vi "test_csm_interface_descp.vi"() -> ()   [LabVIEW 2020]
uses:
  <userlib>/_NEVSTOP/Communicable State Machine(CSM)/_csmHelper/Typedef/Def-Argument Info.ctl
  4ae7eefc-6eeb-4361-9ef0-93d6dbb219bf.vi
  7e83fb4a-f3b1-4b26-86b0-b5537b9c493b.vi
  c018c89d-e81b-45ce-a165-17f998cd6f52.vi
  0c561034-f44a-4e92-a6ab-5fccff993fa6.vi
  <userlib>/_NEVSTOP/Communicable State Machine(CSM)/_Support/Common/Format Timestamp.vi
  <userlib>/_NEVSTOP/Communicable State Machine(CSM)/AdvanceAPI/CSM - Break Down Multiple States String.vi
  <userlib>/_NEVSTOP/Communicable State Machine(CSM)/AdvanceAPI/CSM - Compact Multiple States.vi
  <userlib>/_NEVSTOP/Communicable State Machine(CSM)/AdvanceAPI/CSM - Keywords.vi
  <userlib>/_NEVSTOP/Communicable State Machine(CSM)/addons/MassData-Parameter/_support/FGV-MassData(lvlibp).vi
  <userlib>/_NEVSTOP/Communicable State Machine(CSM)/addons/API-String-Arugments-Support/_Support/Convert API String Arguments to Data(variant).vi
  <userlib>/_NEVSTOP/Communicable State Machine(CSM)/_Shared/Trim Single-line Text.vi
  <userlib>/_NEVSTOP/Communicable State Machine(CSM)/_csmHelper/API/Create From VI Reference.vi
  <userlib>/_NEVSTOP/Communicable State Machine(CSM)/_csmHelper/API/Get All API Interface Info.vi
  <userlib>/_NEVSTOP/Communicable State Machine(CSM)/_csmHelper/API/Get All Status Interface Info.vi
  <userlib>/_NEVSTOP/Communicable State Machine(CSM)/_csmHelper/API/Destroy.vi
  <userlib>/_NEVSTOP/Communicable State Machine(CSM)/_csmHelper/CSM-Helper.lvclass
  <userlib>/_NEVSTOP/Communicable State Machine(CSM)/Communicable State Machine.lvlib
  _support/CSM Mermaid Support.lvlib
panel:
  out "ms":u32
  out "Array 4":cluster{string, "Argument":T1}[](array[cluster])
  out "Array":string[](array[string])
  out "resulting string":string
  out "State History":string
  out "Array 3":cluster{string, "Array":T1[], "Response":T1[]}[](array[cluster])
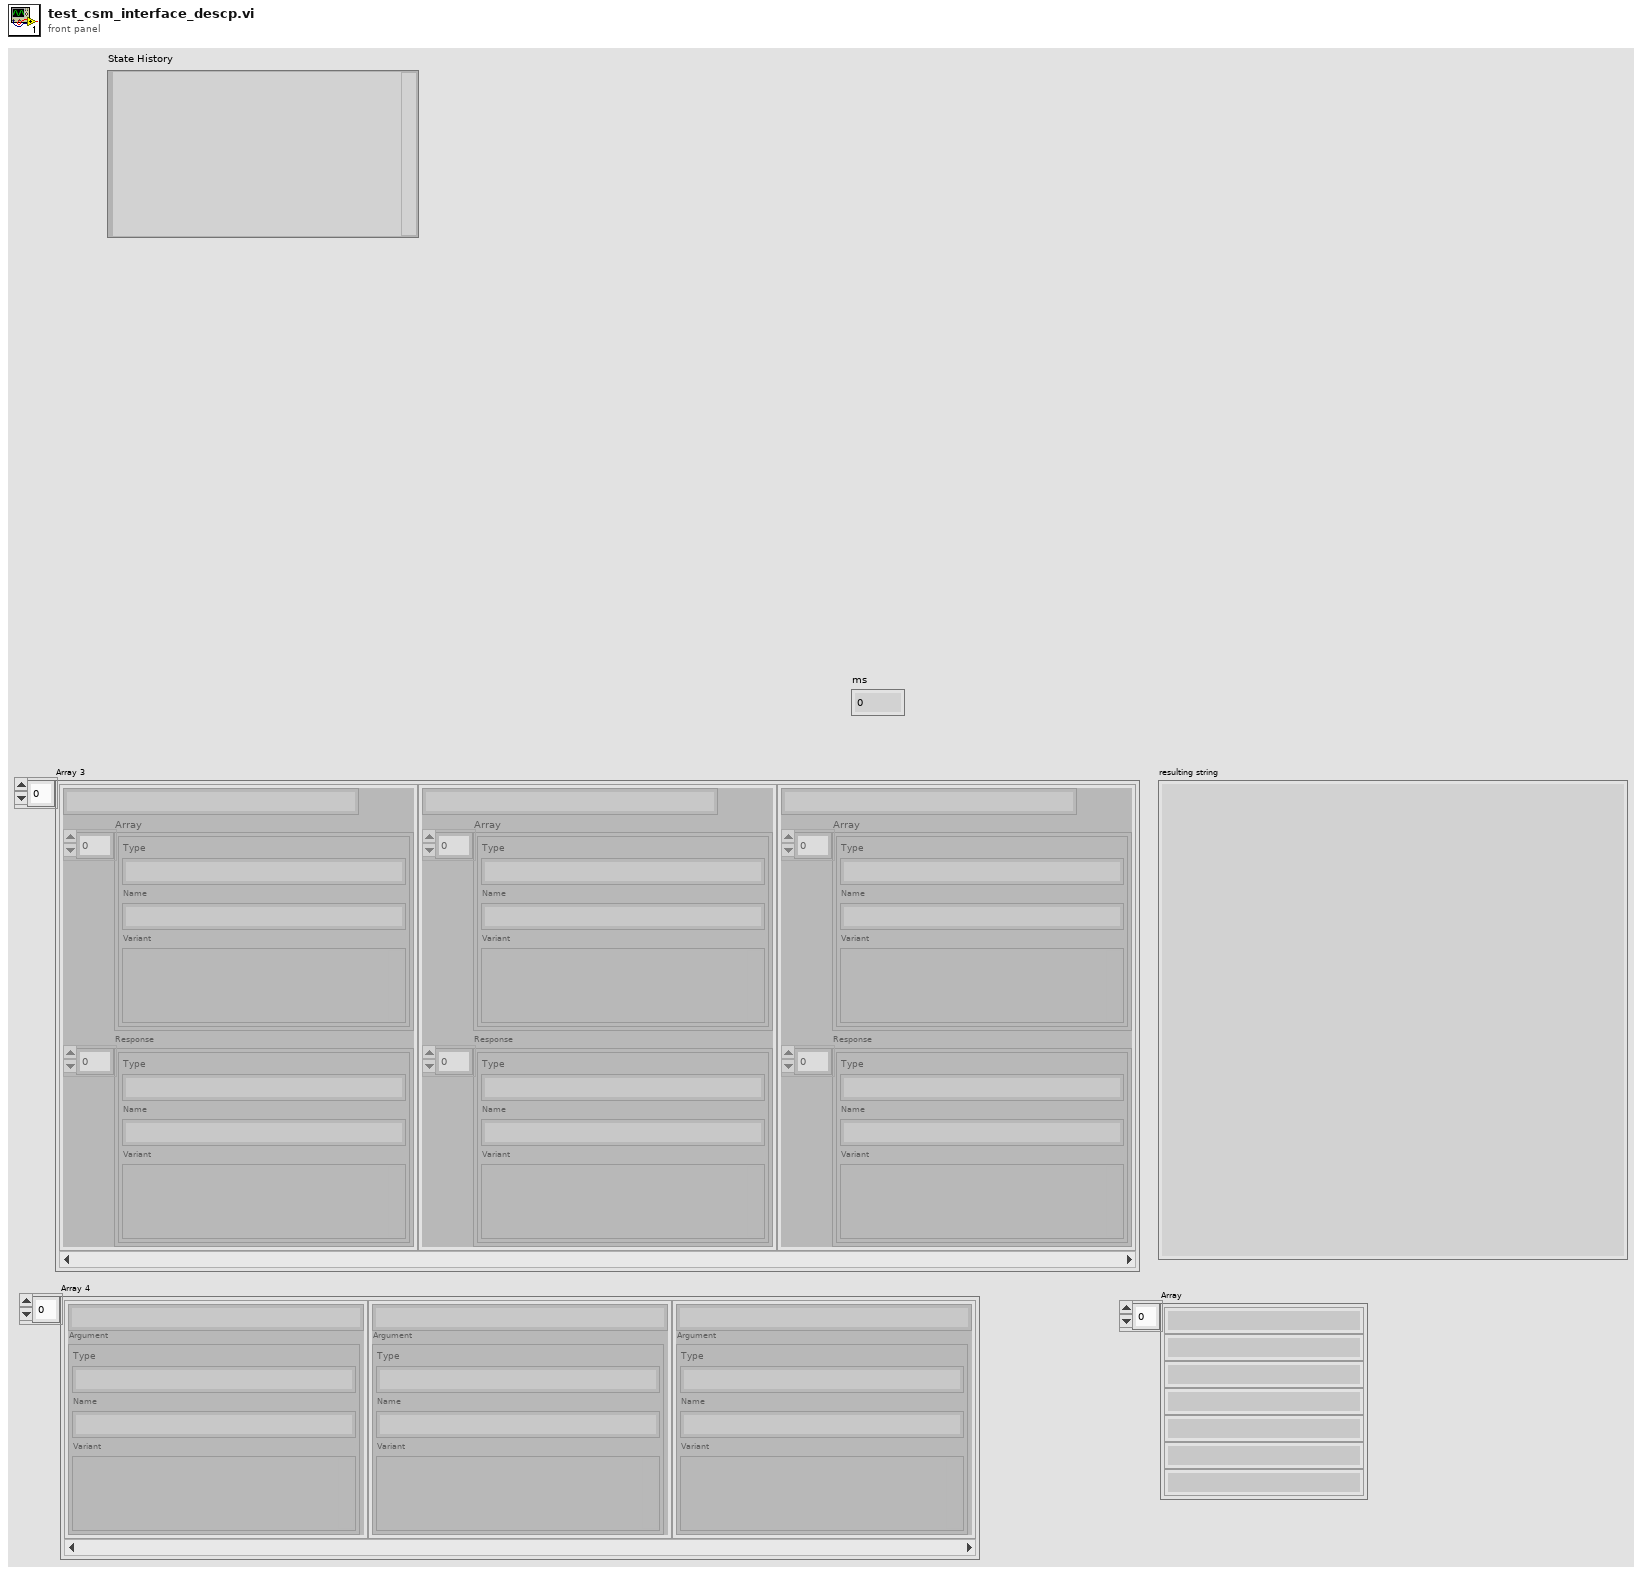
[diagram p1: front panel]
types:
  T1 = typedef "CSM-Helper.lvclass/Def-Argument Info.ctl" = cluster{"Type":string, "Name":string, "Variant":variant}
  T2 = enum32{"Invalid", "Standard", "Closed", "Hidden", "Minimized", "Maximized"}
  T3 = enum32{"invalid app kind", "Development System", "Run Time System", "Student Edition", "Embedded LabVIEW", "Evaluation", "Custom"}
  T4 = typedef "Communicable State Machine.lvlib/_CSM_Response Source Message.ctl" = cluster{"‘State":string, "’Arguments":string, "’Error":errorcluster}
  T5 = cluster{"Core":cluster{"Current VI Reference":refnum<vi>, "Close Panel on Exit?":bool}, "Your Boolean data":bool, "Your string data":string}
  T6 = cluster{"Current VI Reference":refnum<vi>, "Close Panel on Exit?":bool}
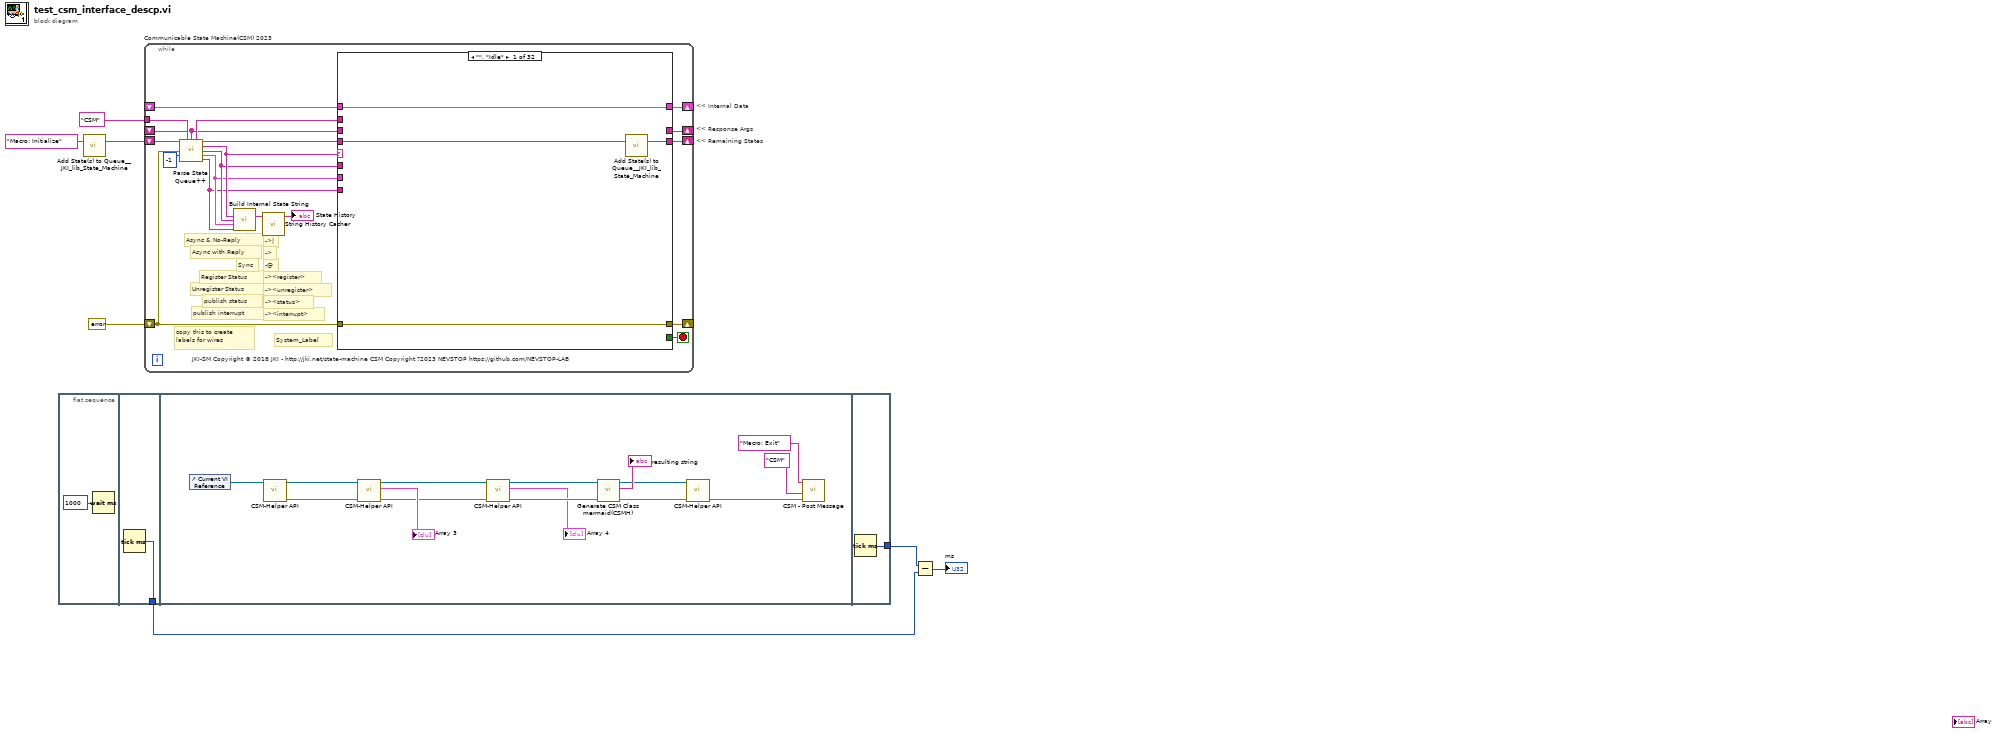
[diagram p0: block diagram]
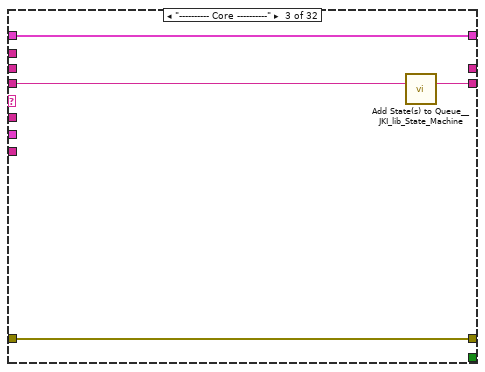
[diagram p3: hidden frame]
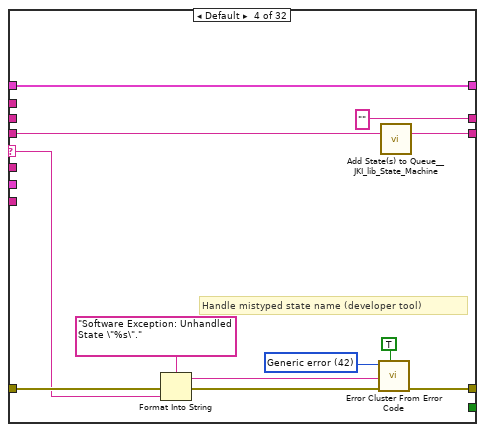
[diagram p4: hidden frame]
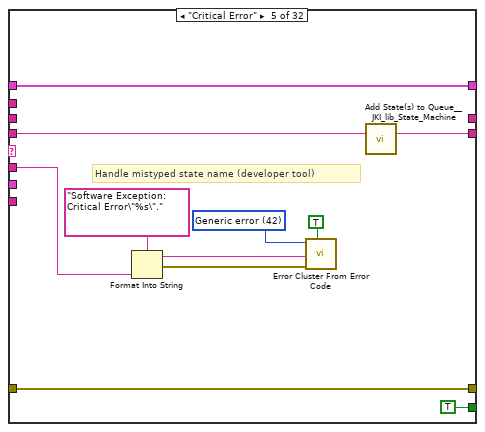
[diagram p5: hidden frame]
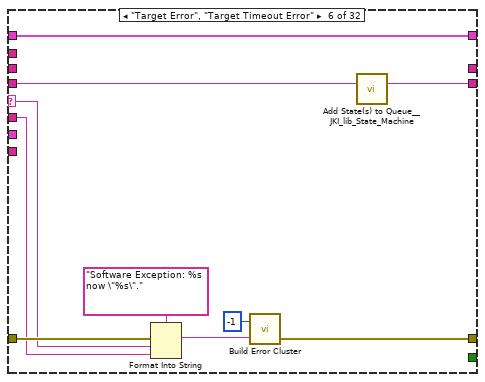
[diagram p6: hidden frame]
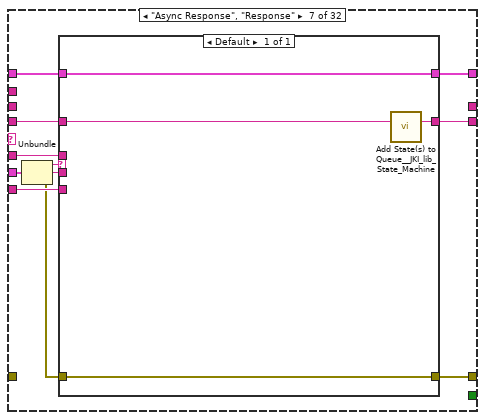
[diagram p7: hidden frame]
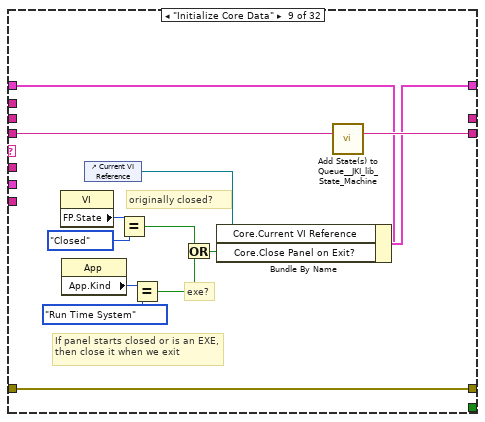
[diagram p9: hidden frame]
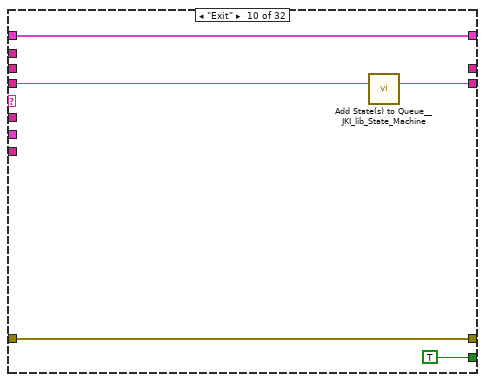
[diagram p10: hidden frame]
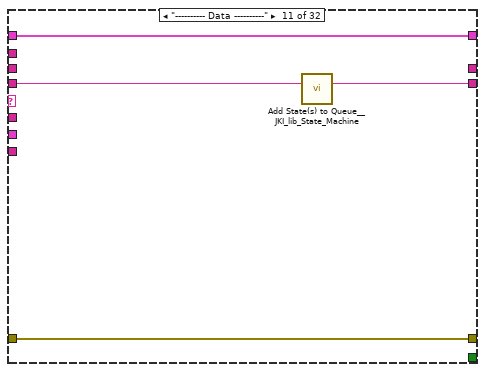
[diagram p11: hidden frame]
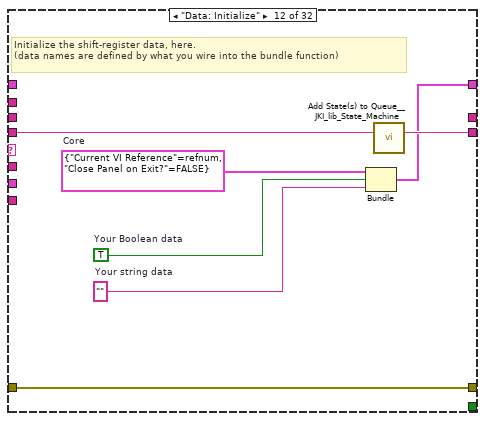
[diagram p12: hidden frame]
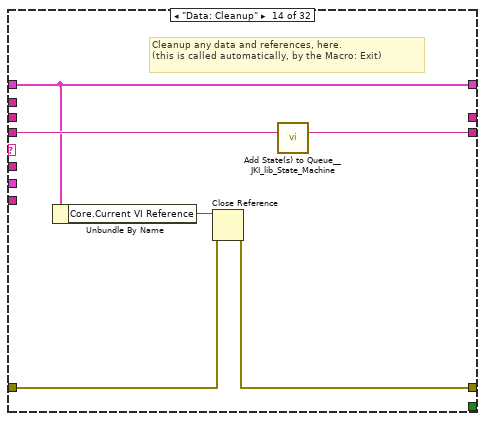
[diagram p14: hidden frame]
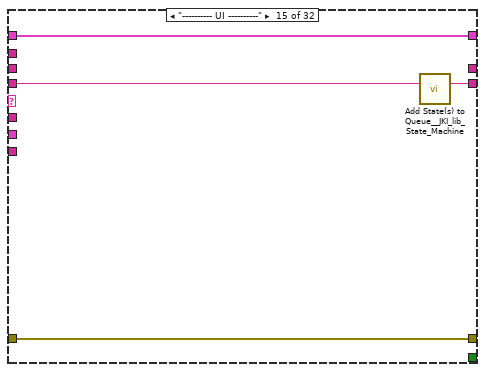
[diagram p15: hidden frame]
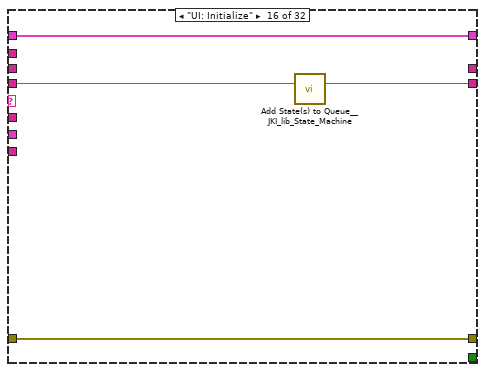
[diagram p16: hidden frame]
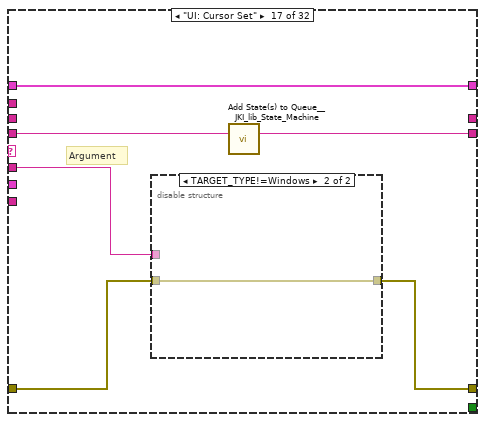
[diagram p17: hidden frame]
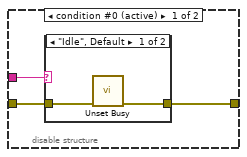
[diagram p18: hidden frame]
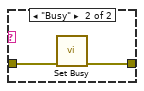
[diagram p19: hidden frame]
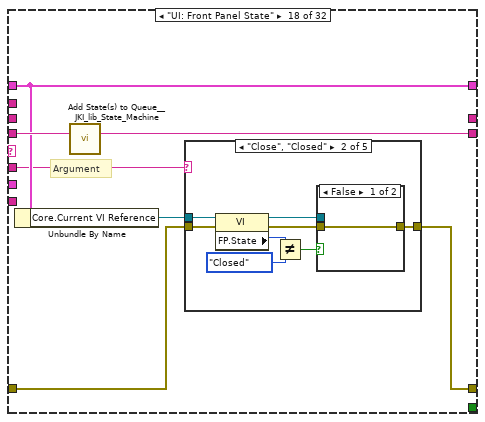
[diagram p20: hidden frame]
diagram:
  # "<< Internal Data"
  # "<< Response Args"
  # "<< Remaining States"
  n1 = flat-sequence {
    tunnel: [w9] -> w2
    tunnel: [w25] -> w3
    frame #0 {
      n2 = Wait (ms)(milliseconds to wait=u32 1000) -> ()  [unwired: 1 out]
    }
    frame #1 {
      n3 = Tick Count (ms)() -> (millisecond timer value=w9:u32)
    }
    frame #2 {
      n4 = control-ref of="Current VI Reference"() -> (w10:refnum<vi>)
      n5 = call-poly <userlib>:"CSM-Helper API.vi"("VI"=w10) -> ("error out"=w24:errorcluster, "CSM-Helper.lvclass"=w22:refnum<class "CSM-Helper.lvclass">)  [unwired: 9 in]
      n6 = call-poly <userlib>:"CSM-Helper API.vi"("error in (no error)"=w24, "CSM-Helper in"=w22) -> ("error out"=w15:errorcluster, "Array"=→"Array 3":cluster{string, "Array":T1[], "Response":T1[]}[], "CSM-Helper out"=w14:refnum<class "CSM-Helper.lvclass">)  [unwired: 7 in]
      n7 = call-poly <userlib>:"CSM-Helper API.vi"("error in (no error)"=w15, "CSM-Helper in"=w14) -> ("error out"=w12:errorcluster, "Array 3"=→"Array 4":cluster{string, "Argument":T1}[], "CSM-Helper out"=w13:refnum<class "CSM-Helper.lvclass">)  [unwired: 7 in]
      n8 = call "Generate CSM Class mermaid(CSMH).vi"("error in (no error)"=w12, "CSM-Helper in"=w13) -> ("error out"=w16:errorcluster, "resulting string"=→"resulting string":string, "CSM-Helper out"=w17:refnum<class "CSM-Helper.lvclass">)  [unwired: 7 in]
      n9 = call-poly <userlib>:"CSM-Helper API.vi"("error in (no error)"=w16, "CSM-Helper in"=w17) -> ("error out"=w21:errorcluster)  [unwired: 8 in, 1 out]
      n10 = call <userlib>:"CSM - Post Message.vi"("Error In (No Error)"=w21, "Target Module"="CSM" ("Name(\"\" to use uuid)"), "State"="Macro: Exit" ("Name(\"\" to use uuid)")) -> ()  [unwired: 8 in, 1 out]
    }
    frame #3 {
      n11 = Tick Count (ms)() -> (millisecond timer value=w25:u32)
    }
  }
  n12 = call <vilib>:"Add State(s) to Queue__JKI_lib_State_Machine.vi"("State(s) in (\"\")"="Macro: Initialize" ("Init State(\"Macro: Initialize\")")) -> ("States Out"=w4:string)  [unwired: 14 in]
  n13 = while "Communicable State Machine(CSM) 2023" {
    shift-right: [w39] -> _
    shift-left: _ -> [w38]
    shift-right: [w42] -> _
    shift-left: errorcluster {"status"=FALSE, "code"=0, "source"=""} ("error out") -> [w37]
    shift-right: [w41] -> _
    shift-left: w4 -> [w43]
    tunnel: "CSM" ("Name(\"\" to use uuid)") -> [w35]
    shift-right: [w36] -> _
    shift-left: _ -> [w27]
    stop <- w40 stop-if-true
    # "-><interrupt>"
    # "-><status>"
    # "-><unregister>"
    # "-><register>"
    # "-@"
    # "->"
    # "->|"
    # "publish interrupt"
    # "publish status"
    # "Unregister Status"
    # "Register Status"
    # "Sync"
    # "Async with Reply"
    # "Async & No-Reply"
    # "copy this to create labels for wires"
    # "System_Label"
    # "JKI-SM Copyright © 2018 JKI - http://jki.net/state-machine CSM Copyright ?2023 NEVSTOP https://github.com/NEVSTOP-LAB"
    n14 = call <userlib>:"Parse State Queue++.vi"("State Queue"=w43, "Name (\"\" to Use UUID)"=w35, "Response Arguments"=w27, "Previous Error"=w37, "Dequeue (1 ms)"=-1 ("Timeout")) -> ("Name Used"=w28:string, "Remaining States"=w44:string, "Current State"=w32:string, "Arguments"=w31:string, "Additional Information"=w30:T4, "Source CSM"=w29:string)  [unwired: 5 in]
    n15 = call <userlib>:"Build Internal State String.vi"("State"=w32, "Arguments (\"\")"=w31, "Additional Information"=w30, "Source (\"\")"=w29) -> ("State With Arguments"=w33:string)  [unwired: 11 in]
    n16 = call <userlib>:"String History Cacher.vi"("String"=w33) -> ("String Cache"=→"State History":string)  [unwired: 10 in]
    n17 = case shown="\"\", \"Idle\"" w32 {
      selector: w32 -> [_ _ _ w57 _ w82 _ _ _ _ _ _ _ _ _ _ _ _ _ _ _ _ _ _ _ _ _ _ _ _ _ _]
      tunnel: w44 -> [w45 w50 w55 w61 w76 w84 w94 w105 w119 w124 w128 w135 w137 w144 w148 w152 w158 w173 w242 w247 w254 w256 w262 w273 w279 w286 w293 w302 w307 w311 w315 w320]
      tunnel: w31 -> [_ _ _ _ w69 w83 w93 _ _ _ _ _ _ _ _ _ w153 w167 _ _ _ _ w263 w270 w277 w284 w288 w300 _ _ _ w319]
      tunnel: w38 -> [w46 w49 w52 w59 w77 w85 w96 w104 w112 w122 w125 _ w136 w139 w145 w150 w156 w169 w239 w244 w251 w255 w264 w272 w278 w285 w292 w301 w304 w308 w312 w323]
      tunnel: [w47 w51 w53 w63 w78 w80 w99 w106 w116 w121 w126 w132 w138 w140 w146 w149 w154 w170 w240 w245 w252 w257 w265 w274 w280 w287 w294 w303 w305 w309 w313 errorcluster {"status"=FALSE, "code"=0, "source"=""} ("error out")] -> w42
      tunnel: w37 -> [w47 w51 w53 w62 w78 w87 _ w106 w116 w121 w126 w132 w138 w141 w146 w149 w155 w171 w240 w245 w252 w257 w265 w274 w280 w287 w294 w303 w305 w309 w313 w321]
      tunnel: [w48 w50 w54 w60 w75 w86 w95 w105 w118 w123 w127 w134 w137 w143 w147 w151 w157 w172 w241 w246 w253 w256 w261 w273 w279 w286 w291 w298 w306 w310 w314 w316] -> w41
      tunnel: [_ _ _ _ TRUE _ _ _ _ TRUE _ _ _ _ _ _ _ _ _ _ _ _ _ _ _ _ _ _ _ _ _ _] -> w40
      tunnel: [w46 w49 w52 w59 w77 w85 w97 w104 w117 w122 w125 w133 w136 w139 w145 w150 w156 w169 w239 w244 w251 w255 w264 w272 w278 w285 w292 w301 w304 w308 w312 w323] -> w39
      tunnel: w29 -> [_ _ _ _ _ _ w91 _ _ _ _ _ _ _ _ _ _ _ _ _ _ _ _ _ _ _ _ _ _ _ _ _]
      tunnel: w30 -> [_ _ _ _ _ _ w98 _ _ _ _ _ _ _ _ _ _ _ _ _ _ _ _ _ _ _ _ _ _ _ _ _]
      tunnel: [_ _ _ "" _ _ _ _ _ _ _ _ _ _ _ _ _ _ _ _ _ _ _ "API1 Response" w276 w283 _ w299 _ _ _ _] -> w36
      tunnel: w28 -> [_ _ _ _ _ _ _ _ _ _ _ _ _ _ _ _ _ _ _ _ _ _ _ _ _ _ _ _ _ _ _ _]
      tunnel: w27 -> [_ _ _ _ _ _ _ _ _ _ _ _ _ _ _ _ _ _ _ _ _ _ _ _ _ _ _ _ _ _ _ _]
      frame "", "Idle" {
        n18 = call <vilib>:"Add State(s) to Queue__JKI_lib_State_Machine.vi"("State(s) in (\"\")"=w45) -> ("States Out"=w48:string)  [unwired: 14 in]
      }
      frame "CSM Documentation" {
      }
      frame "---------- Core ----------" {
        n19 = call <vilib>:"Add State(s) to Queue__JKI_lib_State_Machine.vi"("State(s) in (\"\")"=w55) -> ("States Out"=w54:string)  [unwired: 14 in]
      }
      frame Default {
        w66 = 42 items=["No error", "Argument error", "Memory is full", "Out of zone", "End of file", "File already open", "Generic file I/O error", "File not found", "File permission error", "Disk is full", "Duplicate path", "Too many files open", "System feature not enabled", "Resource file not found", "Cannot add resource", "Resource not found", "Image not found", "Image memory error", "Pen does not exist", "Config type invalid", "Config token not found", "Config parse error", "Config memory error", "Bad external code format", "Bad external code offset", "External code not present", "Null window", "Destroy window error", "Null menu", "Print aborted", "Bad print record", "Print driver error", "Windows error during printing", "Memory error during printing", "Print dialog error", "Generic print error", "Invalid device refnum", "Device not found", "Device parameter error", "Device unit error", "Cannot open device", "Device call aborted", "Generic error", "Cancelled by user", "Object ID too low", "Object ID too high", "Object not in heap", "Unknown heap", "Unknown object (invalid DefProc)", "Unknown object (DefProc not in table)", "Message out of range", "Invalid (null) method", "Unknown message", "Manager call not supported", "Bad address", "Network operation in progress", "Network operation timed out", "Connection is busy", "Network attribute not supported", "Network error", "Address in use", "System out of memory", "Connection aborted", "Connection refused", "Not connected", "Already connected", "Connection closed", "Initialization error (interapplication manager)", "Bad occurrence", "Wait on unbound occurrence handler", "Occurrence queue overflow", "Datalog type conflict", "Unused", "Unrecognized type (interapplication manager)", "Memory corrupt", "Failed to make temporary DLL", "Old CIN version", "Drag socket not found", "Failed to load drop-object", "Failed to register OLE object", "Failed to release OLE object", "Format specifier type mismatch", "Unknown format specifier", "Too few format specifiers", "Too many format specifiers", "Scan failed", "Newer CIN version", "Error converting to variant", "Runtime menu error", "Password tampered", "Variant attribute not found", "Incompatible variant data type", "Event data is not available", "Event Store is not present", "Occurrence is not found", "Event Queue is not created", "Event info is not available", "Refnum passed is NULL", "Error retrieving Class GUID", "Error retrieving CoClass GUID", "Error retrieving TypeLib GUID.", "Bad built application magic bytes.", "Specific driver is different from the specific driver associated with the Logical Name.", "There is no session opened to the class driver.", "Max Error", "MAX - Error with config objects", "MAX - Error loading configuration", "MAX - Group not supported"]
        # "Handle mistyped state name (developer tool)"
        n20 = Format Into String(format string="Software Exception: Unhandled State \"%s\"." ("message"), error in=w62, w57) -> (resulting string=w65:string, error out=w64:errorcluster)  [unwired: 1 in]
        n21 = call <vilib>:"Error Cluster From Error Code.vi"("show call chain? (False)"=TRUE, "error in (no error)"=w64, "error message (\"\")"=w65, "error code (0)"=w66) -> ("error out"=w63:errorcluster)  [unwired: 5 in]
        n22 = call <vilib>:"Add State(s) to Queue__JKI_lib_State_Machine.vi"("State(s) in (\"\")"=w61) -> ("States Out"=w60:string)  [unwired: 14 in]
      }
      frame "Critical Error" {
        w73 = 42 items=["No error", "Argument error", "Memory is full", "Out of zone", "End of file", "File already open", "Generic file I/O error", "File not found", "File permission error", "Disk is full", "Duplicate path", "Too many files open", "System feature not enabled", "Resource file not found", "Cannot add resource", "Resource not found", "Image not found", "Image memory error", "Pen does not exist", "Config type invalid", "Config token not found", "Config parse error", "Config memory error", "Bad external code format", "Bad external code offset", "External code not present", "Null window", "Destroy window error", "Null menu", "Print aborted", "Bad print record", "Print driver error", "Windows error during printing", "Memory error during printing", "Print dialog error", "Generic print error", "Invalid device refnum", "Device not found", "Device parameter error", "Device unit error", "Cannot open device", "Device call aborted", "Generic error", "Cancelled by user", "Object ID too low", "Object ID too high", "Object not in heap", "Unknown heap", "Unknown object (invalid DefProc)", "Unknown object (DefProc not in table)", "Message out of range", "Invalid (null) method", "Unknown message", "Manager call not supported", "Bad address", "Network operation in progress", "Network operation timed out", "Connection is busy", "Network attribute not supported", "Network error", "Address in use", "System out of memory", "Connection aborted", "Connection refused", "Not connected", "Already connected", "Connection closed", "Initialization error (interapplication manager)", "Bad occurrence", "Wait on unbound occurrence handler", "Occurrence queue overflow", "Datalog type conflict", "Unused", "Unrecognized type (interapplication manager)", "Memory corrupt", "Failed to make temporary DLL", "Old CIN version", "Drag socket not found", "Failed to load drop-object", "Failed to register OLE object", "Failed to release OLE object", "Format specifier type mismatch", "Unknown format specifier", "Too few format specifiers", "Too many format specifiers", "Scan failed", "Newer CIN version", "Error converting to variant", "Runtime menu error", "Password tampered", "Variant attribute not found", "Incompatible variant data type", "Event data is not available", "Event Store is not present", "Occurrence is not found", "Event Queue is not created", "Event info is not available", "Refnum passed is NULL", "Error retrieving Class GUID", "Error retrieving CoClass GUID", "Error retrieving TypeLib GUID.", "Bad built application magic bytes.", "Specific driver is different from the specific driver associated with the Logical Name.", "There is no session opened to the class driver.", "Max Error", "MAX - Error with config objects", "MAX - Error loading configuration", "MAX - Group not supported"]
        # "Handle mistyped state name (developer tool)"
        n23 = Format Into String(format string="Software Exception: Critical Error\"%s\"." ("message"), w69) -> (resulting string=w72:string, error out=w71:errorcluster)  [unwired: 2 in]
        n24 = call <vilib>:"Error Cluster From Error Code.vi"("show call chain? (False)"=TRUE, "error in (no error)"=w71, "error message (\"\")"=w72, "error code (0)"=w73) -> ()  [unwired: 5 in, 1 out]
        n25 = call <vilib>:"Add State(s) to Queue__JKI_lib_State_Machine.vi"("State(s) in (\"\")"=w76) -> ("States Out"=w75:string)  [unwired: 14 in]
      }
      frame "Target Error", "Target Timeout Error" {
        n26 = Format Into String(format string="Software Exception: %s now \"%s\"." ("message"), error in=w87, w82, w83) -> (resulting string=w81:string)  [unwired: 1 in, 1 out]
        n27 = call <userlib>:"Build Error Cluster.vi"("String to Prepend to Source (\"\")"=w81, "Code"=-1 ("code")) -> ("error out"=w80:errorcluster)
        n28 = call <vilib>:"Add State(s) to Queue__JKI_lib_State_Machine.vi"("State(s) in (\"\")"=w84) -> ("States Out"=w86:string)  [unwired: 14 in]
      }
      frame "Async Response", "Response" {
        n29 = Unbundle(w98) -> ("‘State"=w92:string, "’Arguments"=w90:string, "’Error"=w89:errorcluster)
        n30 = case shown="Default" w92 {
          tunnel: [w103] -> w99
          tunnel: w89 -> [w103]
          tunnel: [w102] -> w97
          tunnel: w96 -> [w102]
          tunnel: [w100] -> w95
          tunnel: w94 -> [w101]
          tunnel: w93 -> [_]
          tunnel: w91 -> [_]
          tunnel: w90 -> [_]
          frame Default {
            n31 = call <vilib>:"Add State(s) to Queue__JKI_lib_State_Machine.vi"("State(s) in (\"\")"=w101) -> ("States Out"=w100:string)  [unwired: 14 in]
          }
        }
      }
      frame "Async Message Posted" {
      }
      frame "Initialize Core Data" {
        # "originally closed?"
        # "exe?"
        # "If panel starts closed or is an EXE, then close it when we exit"
        n32 = property class="VI"() -> ("FP.State"=w109:T2)  [unwired: 2 in, 2 out]
        n33 = property class="App"() -> ("App.Kind"=w115:T3)  [unwired: 2 in, 2 out]
        n34 = control-ref of="Current VI Reference"() -> (w110:refnum<vi>)
        n35 = Equal?(x=w109, y=T2."Closed" ("Front Panel Window:State")) -> (x = y?=w107:bool)
        n36 = Equal?(x=w115, y=T3."Run Time System" ("Application:Kind")) -> (x = y?=w113:bool)
        n37 = Or(x=w107, y=w113) -> (x .or. y?=w111:bool)
        n38 = Bundle By Name(cluster=w112, "Core.Current VI Reference"=w110, "Core.Close Panel on Exit?"=w111) -> (w117:T5)
        n39 = call <vilib>:"Add State(s) to Queue__JKI_lib_State_Machine.vi"("State(s) in (\"\")"=w119) -> ("States Out"=w118:string)  [unwired: 14 in]
      }
      frame "Exit" {
        n40 = call <vilib>:"Add State(s) to Queue__JKI_lib_State_Machine.vi"("State(s) in (\"\")"=w124) -> ("States Out"=w123:string)  [unwired: 14 in]
      }
      frame "---------- Data ----------" {
        n41 = call <vilib>:"Add State(s) to Queue__JKI_lib_State_Machine.vi"("State(s) in (\"\")"=w128) -> ("States Out"=w127:string)  [unwired: 14 in]
      }
      frame "Data: Initialize" {
        w129 = T6 {"Current VI Reference"=refnum, "Close Panel on Exit?"=FALSE}  # Core
        w131 = TRUE  # Your Boolean data
        w130 = ""  # Your string data
        # "Initialize the shift-register data, here.\n(data names are defined by what you wire into the bundle function)"
        n42 = Bundle("Core"=w129, "Your Boolean data"=w131, "Your string data"=w130) -> (w133:T5)  [unwired: 1 in]
        n43 = call <vilib>:"Add State(s) to Queue__JKI_lib_State_Machine.vi"("State(s) in (\"\")"=w135) -> ("States Out"=w134:string)  [unwired: 14 in]
      }
      frame "Data: Update Indicators" {
      }
      frame "Data: Cleanup" {
        # "Cleanup any data and references, here.\n(this is called automatically, by the Macro: Exit)"
        n44 = Unbundle By Name(w139) -> ("Core.Current VI Reference"=w142:refnum<vi>)
        n45 = Close Reference(reference=w142, error in (no error)=w141) -> (error out=w140:errorcluster)
        n46 = call <vilib>:"Add State(s) to Queue__JKI_lib_State_Machine.vi"("State(s) in (\"\")"=w144) -> ("States Out"=w143:string)  [unwired: 14 in]
      }
      frame "---------- UI ----------" {
        n47 = call <vilib>:"Add State(s) to Queue__JKI_lib_State_Machine.vi"("State(s) in (\"\")"=w148) -> ("States Out"=w147:string)  [unwired: 14 in]
      }
      frame "UI: Initialize" {
        n48 = call <vilib>:"Add State(s) to Queue__JKI_lib_State_Machine.vi"("State(s) in (\"\")"=w152) -> ("States Out"=w151:string)  [unwired: 14 in]
      }
      frame "UI: Cursor Set" {
        # "Argument"
        n49 = disable-structure shown="TARGET_TYPE!=Windows" {
          disable-tunnel: w155 -> [w161 w166]
          disable-tunnel: [w160 w166] -> w154
          disable-tunnel: w153 -> [w159 _]
          frame condition #0 (active) {
            n50 = case shown="\"Idle\", Default" w159 {
              tunnel: w161 -> [w163 w165]
              tunnel: [w162 w164] -> w160
              frame "Idle", Default {
                n51 = call <vilib>:"Unset Busy.vi"("error in (no error)"=w163) -> ("error out"=w162:errorcluster)  [unwired: 10 in]
              }
              frame "Busy" {
                n52 = call <vilib>:"Set Busy.vi"("error in (no error)"=w165) -> ("error out"=w164:errorcluster)  [unwired: 9 in, 1 out]
              }
            }
          }
          frame condition #1 {
          }
        }
        n53 = call <vilib>:"Add State(s) to Queue__JKI_lib_State_Machine.vi"("State(s) in (\"\")"=w158) -> ("States Out"=w157:string)  [unwired: 14 in]
      }
      frame "UI: Front Panel State" {
        # "Argument"
        n54 = Unbundle By Name(w169) -> ("Core.Current VI Reference"=w168:refnum<vi>)
        n55 = call <vilib>:"Add State(s) to Queue__JKI_lib_State_Machine.vi"("State(s) in (\"\")"=w173) -> ("States Out"=w172:string)  [unwired: 14 in]
        n56 = case shown="\"Close\", \"Closed\"" w167 {
          tunnel: w171 -> [w179 w194 w205 w218 w231]
          tunnel: [w181 w195 w207 w220 w233] -> w170
          tunnel: w168 -> [w180 w192 w206 w219 w232]
          frame "Open", "Standard", Default {
            w174 = T2."Standard" ("State")
            n57 = property class="VI"(reference=w180, error in=w179) -> (reference out=w177:refnum<vi>, error out=w178:errorcluster, "FP.State"=w176:T2)
            n58 = Not Equal?(x=w176, y=w174) -> (x != y?=w175:bool)
            n59 = case shown="True" w175 {
              tunnel: [w185 w187] -> w181
              tunnel: w178 -> [w184 w187]
              tunnel: w177 -> [w183 _]
              tunnel: w174 -> [w182 _]
              frame True {
                n60 = invoke class="VI" method="FP.Open"(reference=w183, error in=w184, "Activate"=TRUE, "State"=w182) -> (error out=w185:errorcluster)  [unwired: 1 in, 4 out]
              }
              frame False {
              }
            }
          }
          frame "Close", "Closed" {
            n61 = property class="VI"(reference=w192, error in=w194) -> (reference out=w191:refnum<vi>, error out=w193:errorcluster, "FP.State"=w189:T2)
            n62 = Not Equal?(x=w189, y=T2."Closed" ("Front Panel Window:State")) -> (x != y?=w188:bool)
            n63 = case shown="False" w188 {
              tunnel: [w196 w199] -> w195
              tunnel: w193 -> [w196 w198]
              tunnel: w191 -> [_ w197]
              frame False {
              }
              frame True {
                n64 = invoke class="VI" method="FP.Close"(reference=w197, error in=w198) -> (error out=w199:errorcluster)  [unwired: 1 in, 2 out]
              }
            }
          }
          frame "Hidden", "Hide" {
            w200 = T2."Hidden" ("State")
            n65 = property class="VI"(reference=w206, error in=w205) -> (reference out=w203:refnum<vi>, error out=w204:errorcluster, "FP.State"=w202:T2)
            n66 = Not Equal?(x=w202, y=w200) -> (x != y?=w201:bool)
            n67 = case shown="True" w201 {
              tunnel: [w211 w212] -> w207
              tunnel: w204 -> [w210 w212]
              tunnel: w203 -> [w209 _]
              tunnel: w200 -> [w208 _]
              frame True {
                n68 = invoke class="VI" method="FP.Open"(reference=w209, error in=w210, "State"=w208) -> (error out=w211:errorcluster)  [unwired: 2 in, 4 out]
              }
              frame False {
              }
            }
          }
          frame "Minimize", "Minimized" {
            w213 = T2."Minimized" ("State")
            n69 = property class="VI"(reference=w219, error in=w218) -> (reference out=w216:refnum<vi>, error out=w217:errorcluster, "FP.State"=w215:T2)
            n70 = Not Equal?(x=w215, y=w213) -> (x != y?=w214:bool)
            n71 = case shown="True" w214 {
              tunnel: [w224 w225] -> w220
              tunnel: w217 -> [w223 w225]
              tunnel: w216 -> [w222 _]
              tunnel: w213 -> [w221 _]
              frame True {
                n72 = invoke class="VI" method="FP.Open"(reference=w222, error in=w223, "State"=w221) -> (error out=w224:errorcluster)  [unwired: 2 in, 4 out]
              }
              frame False {
              }
            }
          }
          frame "Maximize", "Maximized" {
            w226 = T2."Maximized" ("State")
            n73 = property class="VI"(reference=w232, error in=w231) -> (reference out=w229:refnum<vi>, error out=w230:errorcluster, "FP.State"=w228:T2)
            n74 = Not Equal?(x=w228, y=w226) -> (x != y?=w227:bool)
            n75 = case shown="True" w227 {
              tunnel: [w237 w238] -> w233
              tunnel: w230 -> [w236 w238]
              tunnel: w229 -> [w235 _]
              tunnel: w226 -> [w234 _]
              frame True {
                n76 = invoke class="VI" method="FP.Open"(reference=w235, error in=w236, "State"=w234) -> (error out=w237:errorcluster)  [unwired: 2 in, 4 out]
              }
              frame False {
              }
            }
          }
        }
      }
      frame "---------- Macro ----------" {
        n77 = call <vilib>:"Add State(s) to Queue__JKI_lib_State_Machine.vi"("State(s) in (\"\")"=w242) -> ("States Out"=w241:string)  [unwired: 14 in]
      }
      frame "Macro: Initialize" {
        n78 = call <vilib>:"Add State(s) to Queue__JKI_lib_State_Machine.vi"("State(s) in Front (\"\")"="Data: Initialize\nInitialize Core Data\nData: Update Indicators", "State(s) in (\"\")"=w247) -> ("States Out"=w246:string)  [unwired: 13 in]
      }
      frame "Macro: Exit" {
        n79 = call <vilib>:"Add State(s) to Queue__JKI_lib_State_Machine.vi"("State(s) in Front (\"\")"="//Exit Sub-Modules ", "State(s) at Back (\"\")"="Data: Cleanup\nExit") -> ("States Out"=w249:string)  [unwired: 13 in]
        n80 = call <vilib>:"Add State(s) to Queue__JKI_lib_State_Machine.vi"("State(s) in Front (\"\")"=w249, "State(s) in (\"\")"=w254) -> ("States Out"=w253:string)  [unwired: 13 in]
      }
      frame "---------- API ----------" {
      }
      frame "API: API3" {
        n81 = case shown="\"a\"" w263 {
          tunnel: [_ w266] -> w258
          frame "b", Default {
          }
          frame "a" {
            n82 = call "CSM - Convert MassData to Argument.vim"("Data"=waveform(dbl) {"t0"=timestamp(0 s since 1904-01-01), "dt"=1.0, "Y"=[]} ("Waveform")) -> ("MassData Argument"=w266:string)  [unwired: 7 in, 1 out]
          }
        }
        n83 = call <vilib>:"Build State String with Arguments__JKI_lib_State_Machine.vi"("Arguments (\"\")"=w258, "State"="status2") -> ("State with Arguments"=w259:string)  [unwired: 4 in]
        n84 = call <userlib>:"CSM - Broadcast Status Change.vi"("Status With Arguments"=w259, "State Queue"=w262) -> ("Remaining States"=w261:string)  [unwired: 13 in]
      }
      frame "API: API1" {
        n85 = call "Convert API String Arguments to Data.vim"("Reference Type"=cluster{"status":bool, "code":i32} {"status"=FALSE, "code"=0} ("error in (no error)"), "API String"=w270) -> ("Data"=w268:cluster{"status":bool, "code":i32})  [unwired: 6 in, 1 out]
        n86 = flat-sequence {
          tunnel: w268 -> [_]
          frame #0 {
          }
        }
      }
      frame "API: API2" {
        # "unpack Hex String  to Variant\nif complex parameter is needed."
        n87 = call <userlib>:"CSM - Convert HexStr to Data.vi"("HEX String"=w277) -> ()  [unwired: 7 in, 2 out]
        n88 = call <userlib>:"CSM - Convert Data to HexStr.vi"("Variant"=0) -> ("HEX String (0-9,A-F)"=w276:string)  [unwired: 8 in]
      }
      frame "API: API4" {
        # "unpack Hex String  to Variant\nif complex parameter is needed."
        n89 = call "CSM - Convert Argument to MassData.vim"("Type"=dbl[] [], "MassData Argument"=w284) -> ("Data"=w282:dbl[])  [unwired: 6 in, 1 out]
        n90 = call "CSM - Convert MassData to Argument.vim"("Data"=w282) -> ("MassData Argument"=w283:string)  [unwired: 7 in, 1 out]
      }
      frame "API: API6" {
        n91 = call <vilib>:"Build State String with Arguments__JKI_lib_State_Machine.vi"("Arguments (\"\")"=w288, "State"="API6 Status" ("Status with Arguments")) -> ("State with Arguments"=w290:string)  [unwired: 4 in]
        n92 = call <userlib>:"CSM - Broadcast Status Change.vi"("Status With Arguments"=w290, "State Queue"=w293) -> ("Remaining States"=w291:string)  [unwired: 13 in]
      }
      frame "API: API5" {
        n93 = call <userlib>:"CSM - Revert Arguments-Safe String.vi"("Safe Argument String"=w300) -> ("Origin Argument String"=w295:string)  [unwired: 8 in]
        n94 = call <vilib>:"Build State String with Arguments__JKI_lib_State_Machine.vi"("Arguments (\"\")"=w295, "State"="API5 Status" ("Status with Arguments")) -> ("State with Arguments"=w297:string)  [unwired: 4 in]
        n95 = call <userlib>:"CSM - Make String Arguments Safe.vi"("Argument String"=w295) -> ("Safe Argument String"=w299:string)  [unwired: 8 in]
        n96 = call <userlib>:"CSM - Broadcast Status Change.vi"("Status With Arguments"=w297, "State Queue"=w302) -> ("Remaining States"=w298:string)  [unwired: 13 in]
      }
      frame "---------- Action ----------" {
        n97 = call <vilib>:"Add State(s) to Queue__JKI_lib_State_Machine.vi"("State(s) in (\"\")"=w307) -> ("States Out"=w306:string)  [unwired: 14 in]
      }
      frame "Action: action1" {
        n98 = call <vilib>:"Add State(s) to Queue__JKI_lib_State_Machine.vi"("State(s) in (\"\")"=w311) -> ("States Out"=w310:string)  [unwired: 14 in]
      }
      frame "Action: action2" {
        n99 = call <vilib>:"Add State(s) to Queue__JKI_lib_State_Machine.vi"("State(s) in (\"\")"=w315) -> ("States Out"=w314:string)  [unwired: 14 in]
      }
      frame "Error Handler" {
        # "Clear error"
        n100 = case shown="Error" w321 {
          selector: w321 -> [_ w330]
          tunnel: [w329 w332] -> w317
          tunnel: w320 -> [w329 w331]
          tunnel: w319 -> [w328 _]
          tunnel: [w327 w330] -> w322
          frame No Error {
            n101 = call <userlib>:"CSM - Convert Argument to Error.vi"("Argument"=w328) -> ("Error"=w327:errorcluster)  [unwired: 4 in]
            n102 = flat-sequence {
              frame #0 {
              }
            }
          }
          frame Error {
            n103 = call <userlib>:"CSM - Convert Error to Argument.vi"("Error"=w330) -> ("Argument"=w334:string)  [unwired: 4 in]
            n104 = call <vilib>:"Build State String with Arguments__JKI_lib_State_Machine.vi"("Arguments (\"\")"=w334, "State"="Error Occurred" ("Status with Arguments")) -> ("State with Arguments"=w333:string)  [unwired: 4 in]
            n105 = call <userlib>:"CSM - Broadcast Status Change.vi"("Status With Arguments"=w333, "State Queue"=w331) -> ("Remaining States"=w332:string)  [unwired: 13 in]
          }
        }
        n106 = disable-structure shown="Enabled" {
          disable-tunnel: w322 -> [w325 w326]
          frame Enabled {
            n107 = call <vilib>:"General Error Handler.vi"("error in (no error)"=w325) -> ()  [unwired: 10 in, 5 out]
          }
          frame Disabled {
            n108 = call <vilib>:"Clear Errors.vi"("error in (no error)"=w326) -> ()  [unwired: 5 in, 2 out]
          }
        }
        n109 = call <vilib>:"Add State(s) to Queue__JKI_lib_State_Machine.vi"("State(s) in Front (\"\")"="// Post Error States", "State(s) in (\"\")"=w317) -> ("States Out"=w316:string)  [unwired: 13 in]
      }
    }
  }
  n110 = Subtract(x=w3, y=w2) -> (x-y=→"ms":u32)
